vi "Showcase.vi"   [LabVIEW 2018]
uses:
  TwinCAT ADS Class/TwinCAT ADS.lvclass
  3dda1637-87fb-4573-9f5a-29747ec08bbd.vi
  cc6a6ab7-5b69-4027-b05b-cb099868c74d.vi
  50ffd016-ed67-41eb-ba02-c9a09dc735e3.vi
panel:
  # "VIs are on the Block Diagram"
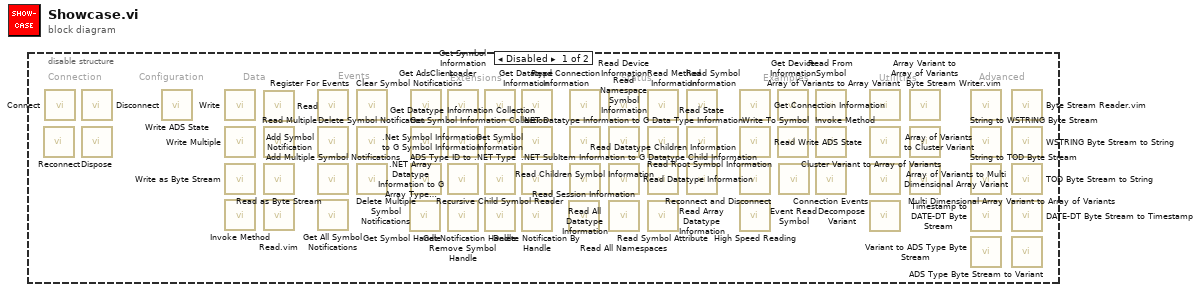
[diagram p0: block diagram]
diagram:
  n1 = disable-structure shown="Disabled" {
    frame Disabled {
      # "Events"
      # "Advanced"
      # "Utilities"
      # "Examples"
      # "Status"
      # "Extensions"
      # "Data"
      # "Configuration"
      # "Connection"
      n2 = call "Reconnect.vi"() -> ()  [unwired: 10 in, 2 out]
      n3 = call "Connect.vi"() -> ()  [unwired: 10 in, 2 out]
      n4 = call "Disconnect.vi"() -> ()  [unwired: 9 in, 3 out]
      n5 = call "Dispose.vi"() -> ()  [unwired: 11 in, 1 out]
      n6 = call "Write ADS State.vi"() -> ()  [unwired: 10 in, 2 out]
      n7 = call "Write.vi"() -> ()  [unwired: 10 in, 2 out]
      n8 = call "Write Multiple.vi"() -> ()  [unwired: 10 in, 2 out]
      n9 = call "Write as Byte Stream.vi"() -> ()  [unwired: 9 in, 3 out]
      n10 = call "Invoke Method.vi"() -> ()  [unwired: 8 in, 4 out]
      n11 = call "Read.vi"() -> ()  [unwired: 9 in, 3 out]
      n12 = call "Read Multiple.vi"() -> ()  [unwired: 9 in, 3 out]
      n13 = call "Read as Byte Stream.vi"() -> ()  [unwired: 9 in, 3 out]
      n14 = call "Read.vim"() -> ()  [unwired: 9 in, 3 out]
      n15 = call "Register For Events.vi"() -> ()  [unwired: 9 in, 3 out]
      n16 = call "Add Symbol Notification.vi"() -> ()  [unwired: 10 in, 2 out]
      n17 = call "Add Multiple Symbol Notifications.vi"() -> ()  [unwired: 10 in, 2 out]
      n18 = call "Get All Symbol Notifications.vi"() -> ()  [unwired: 9 in, 3 out]
      n19 = call "Clear Symbol Notifications.vi"() -> ()  [unwired: 10 in, 2 out]
      n20 = call "Delete Symbol Notification.vi"() -> ()  [unwired: 10 in, 2 out]
      n21 = call "Delete Multiple Symbol Notifications.vi"() -> ()  [unwired: 10 in, 2 out]
      n22 = call "Get Symbol Handle.vi"() -> ()  [unwired: 9 in, 3 out]
      n23 = call "Get AdsClient.vi"() -> ()  [unwired: 9 in, 3 out]
      n24 = call "Get Symbol Information Collection.vi"() -> ()  [unwired: 9 in, 3 out]
      n25 = call "ADS Type ID to .NET Type.vi"() -> ()  [unwired: 9 in, 3 out]
      n26 = call "Get Symbol Information Loader.vi"() -> ()  [unwired: 9 in, 3 out]
      n27 = call "Get Datatype Information Collection.vi"() -> ()  [unwired: 9 in, 3 out]
      n28 = call ".NET Array Datatype Information to G Array Type Information.vi"() -> ()  [unwired: 9 in, 3 out]
      n29 = call "Remove Symbol Handle.vi"() -> ()  [unwired: 10 in, 2 out]
      n30 = call "Get Symbol Information.vi"() -> ()  [unwired: 9 in, 3 out]
      n31 = call ".Net Symbol Information to G Symbol Information.vi"() -> ()  [unwired: 8 in, 3 out]
      n32 = call "Recursive Child Symbol Reader.vi"() -> ()  [unwired: 9 in, 3 out]
      n33 = call "Get Notification Handle.vi"() -> ()  [unwired: 9 in, 3 out]
      n34 = call "Get Datatype Information.vi"() -> ()  [unwired: 9 in, 3 out]
      n35 = call ".NET Datatype Information to G Data Type Information.vi"() -> ()  [unwired: 9 in, 3 out]
      n36 = call ".NET SubItem Information to G Datatype Child Information.vi"() -> ()  [unwired: 9 in, 3 out]
      n37 = call "Delete Notification By Handle.vi"() -> ()  [unwired: 10 in, 2 out]
      n38 = call "Read Session Information.vi"() -> ()  [unwired: 9 in, 3 out]
      n39 = call "Read Connection Information.vi"() -> ()  [unwired: 9 in, 3 out]
      n40 = call "Read Children Symbol Information.vi"() -> ()  [unwired: 9 in, 3 out]
      n41 = call "Read All Datatype Information.vi"() -> ()  [unwired: 9 in, 3 out]
      n42 = call "Read Device Information.vi"() -> ()  [unwired: 9 in, 3 out]
      n43 = call "Read Namespace Symbol Information.vi"() -> ()  [unwired: 9 in, 3 out]
      n44 = call "Read Datatype Information.vi"() -> ()  [unwired: 9 in, 3 out]
      n45 = call "Read All Namespaces.vi"() -> ()  [unwired: 9 in, 3 out]
      n46 = call "Read Method Information.vi"() -> ()  [unwired: 9 in, 3 out]
      n47 = call "Read Root Symbol Information.vi"() -> ()  [unwired: 9 in, 3 out]
      n48 = call "Read Datatype Children Information.vi"() -> ()  [unwired: 9 in, 3 out]
      n49 = call "Read Symbol Attribute.vi"() -> ()  [unwired: 9 in, 3 out]
      n50 = call "Read Symbol Information.vi"() -> ()  [unwired: 9 in, 3 out]
      n51 = call "Read State.vi"() -> ()  [unwired: 9 in, 3 out]
      n52 = call "Read Array Datatype Information.vi"() -> ()  [unwired: 9 in, 3 out]
      n53 = call "Get Connection Information.vi"() -> ()  [unwired: 12 in]
      n54 = call "Read Write ADS State.vi"() -> ()  [unwired: 12 in]
      n55 = call "Reconnect and Disconnect.vi"() -> ()  [unwired: 12 in]
      n56 = call "High Speed Reading.vi"() -> ()  [unwired: 12 in]
      n57 = call "Get Device Information.vi"() -> ()  [unwired: 12 in]
      n58 = call "Write To Symbol.vi"() -> ()  [unwired: 12 in]
      n59 = call "Event Read Symbol.vi"() -> ()  [unwired: 12 in]
      n60 = call "Read From Symbol.vi"() -> ()  [unwired: 12 in]
      n61 = call "Invoke Method.vi"() -> ()  [unwired: 12 in]
      n62 = call "Connection Events.vi"() -> ()  [unwired: 12 in]
      n63 = call "Array of Variants to Array Variant.vi"() -> ()  [unwired: 10 in, 2 out]
      n64 = call "Array of Variants to Cluster Variant.vi"() -> ()  [unwired: 10 in, 2 out]
      n65 = call "Array of Variants to Multi Dimensional Array Variant.vi"() -> ()  [unwired: 10 in, 2 out]
      n66 = call "Decompose Variant.vi"() -> ()  [unwired: 10 in, 2 out]
      n67 = call "Array Variant to Array of Variants.vi"() -> ()  [unwired: 10 in, 2 out]
      n68 = call "Cluster Variant to Array of Variants.vi"() -> ()  [unwired: 10 in, 2 out]
      n69 = call "Multi Dimensional Array Variant to Array of Variants.vi"() -> ()  [unwired: 10 in, 2 out]
      n70 = call "Byte Stream Writer.vim"() -> ()  [unwired: 10 in, 2 out]
      n71 = call "String to WSTRING Byte Stream.vi"() -> ()  [unwired: 10 in, 2 out]
      n72 = call "String to TOD Byte Stream.vi"() -> ()  [unwired: 10 in, 2 out]
      n73 = call "Timestamp to DATE-DT Byte Stream.vi"() -> ()  [unwired: 10 in, 2 out]
      n74 = call "Variant to ADS Type Byte Stream.vi"() -> ()  [unwired: 9 in, 3 out]
      n75 = call "Byte Stream Reader.vim"() -> ()  [unwired: 10 in, 2 out]
      n76 = call "WSTRING Byte Stream to String.vi"() -> ()  [unwired: 10 in, 2 out]
      n77 = call "TOD Byte Stream to String.vi"() -> ()  [unwired: 10 in, 2 out]
      n78 = call "DATE-DT Byte Stream to Timestamp.vi"() -> ()  [unwired: 10 in, 2 out]
      n79 = call "ADS Type Byte Stream to Variant.vi"() -> ()  [unwired: 9 in, 3 out]
    }
    frame Enabled {
    }
  }
